vi "Main_DataSave.vi"(8 "error in":errorcluster, 11 "Queues in":T1) -> (0 "error out":errorcluster)   [LabVIEW 2019]
uses:
  Queue/TypeDef/#TypeDef_App_Queues.ctl
  User Interface/TypeDef/#TypeDef_Enum_Buttons.ctl
  User Interface/TypeDef/#TypeDef_EventStructureConstant.ctl
  User Interface/TypeDef/#TypeDef_Enum_EventStructure.ctl
  Queue/TypeDef/#TypeDef_NetworkStream.ctl
  Communication/TypeDef/#TypeDef_FromMRtoPC.ctl
  Communication/TypeDef/#TypeDef_FromPCtoMR.ctl
  Communication/TypeDef/#TypeDef_Command.ctl
  Communication/TypeDef/#TypeDef_ErrorHandler_prop.ctl
  Communication/TypeDef/#TypeDef_PropGraph.ctl
  Communication/TypeDef/#TypeDef_PropertiesToSave.ctl
  <vilib>/addons/database/Connection.llb/Conn ObjectReference.ctl
  Test/TypeDef/#TypeDef_DataToTest.ctl
  TypeDef/#TypeDef_EnumOp_DataSaving.ctl
  Communication/TypeDef/#TypeDef_SetGet.ctl
  <vilib>/event_ctls.llb/usereventprio.ctl
  <vilib>/addons/database/NI_Database_API.lvlib
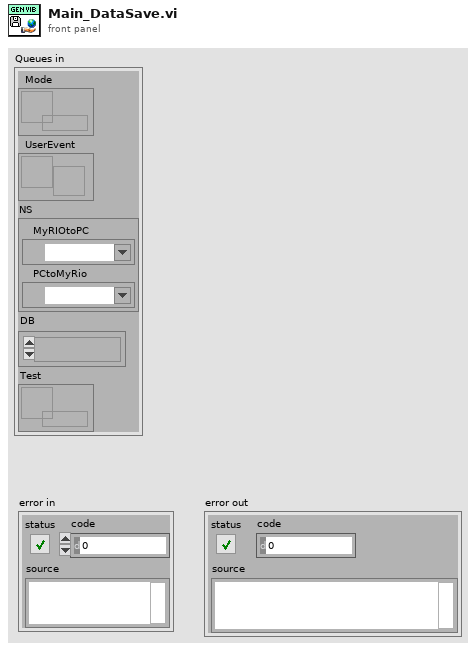
[diagram p1: front panel]
types:
  T1 = typedef "#TypeDef_App_Queues.ctl" = cluster{"Mode":refnum<queue>, "UserEvent":refnum<user-event>, "NS":T2, "DB":T3, "Test":refnum<queue>}
  T2 = typedef "#TypeDef_NetworkStream.ctl" = cluster{"MyRIOtoPC":refnum<k21>, "PCtoMyRio":refnum<k21>}
  T3 = typedef "NI_Database_API.lvlib/Conn ObjectReference.ctl" = refnum<k1>
  T4 = typedef "#TypeDef_FromMRtoPC.ctl" = cluster{"Accessibility":T5, "PropGraph":T8, "No Data?":bool, "WaveformData":waveform(dbl)[]}
  T5 = typedef "#TypeDef_FromPCtoMR.ctl" = cluster{"Command":T6, "Error?":bool, "Stop":bool, "StopPomiar":bool, "Name":string, "FilesPath":path, "ErrorHandler":T7, "Fs":dbl}
  T6 = typedef "#TypeDef_Command.ctl" = enum16{"Start", "End"}
  T7 = typedef "#TypeDef_ErrorHandler_prop.ctl" = cluster{"Threads":enum16{"Acquisistion", "Data Operation", "Save File"}, "ClearError":bool, "Error Out ":errorcluster, "Error":bool}
  T8 = typedef "#TypeDef_PropGraph.ctl" = cluster{"Raw Data":dbl[][], "Poperties":T9, "Power Spectrum / PSD":cluster{"f0":dbl, "df":dbl, "magnitude":dbl[]}[]}
  T9 = typedef "#TypeDef_PropertiesToSave.ctl" = cluster{"RMS values":dbl[], "Max":dbl[], "Min":dbl[], "A(8)":dbl[], "t":dbl, "A(8) Axis":dbl, "Aw":dbl[], "Ak 30min":dbl, "Ak_axis":i32, "Spec":cluster{"f0":dbl, "df":dbl, "magnitude":dbl[]}[]}
  T10 = typedef "#TypeDef_EnumOp_DataSaving.ctl" = enum16{"Idle", "Init", "Collecting", "Saving", "Deleting", "Error_Shutdown", "ClearError"}
  T11 = typedef "#TypeDef_SetGet.ctl" = enum16{"Set", "Get"}
  T12 = enum16{"open", "open or create", "create or replace", "create", "open (read-only)"}
  T13 = typedef "usereventprio.ctl" = enum32{"high priority", "normal priority"}
  T14 = typedef "#TypeDef_Enum_EventStructure.ctl" = enum16{"Default", "Final Items", "Moment Items", "DB"}
  T15 = typedef "#TypeDef_EventStructureConstant.ctl" = cluster{"Value":variant, "Property":T14}
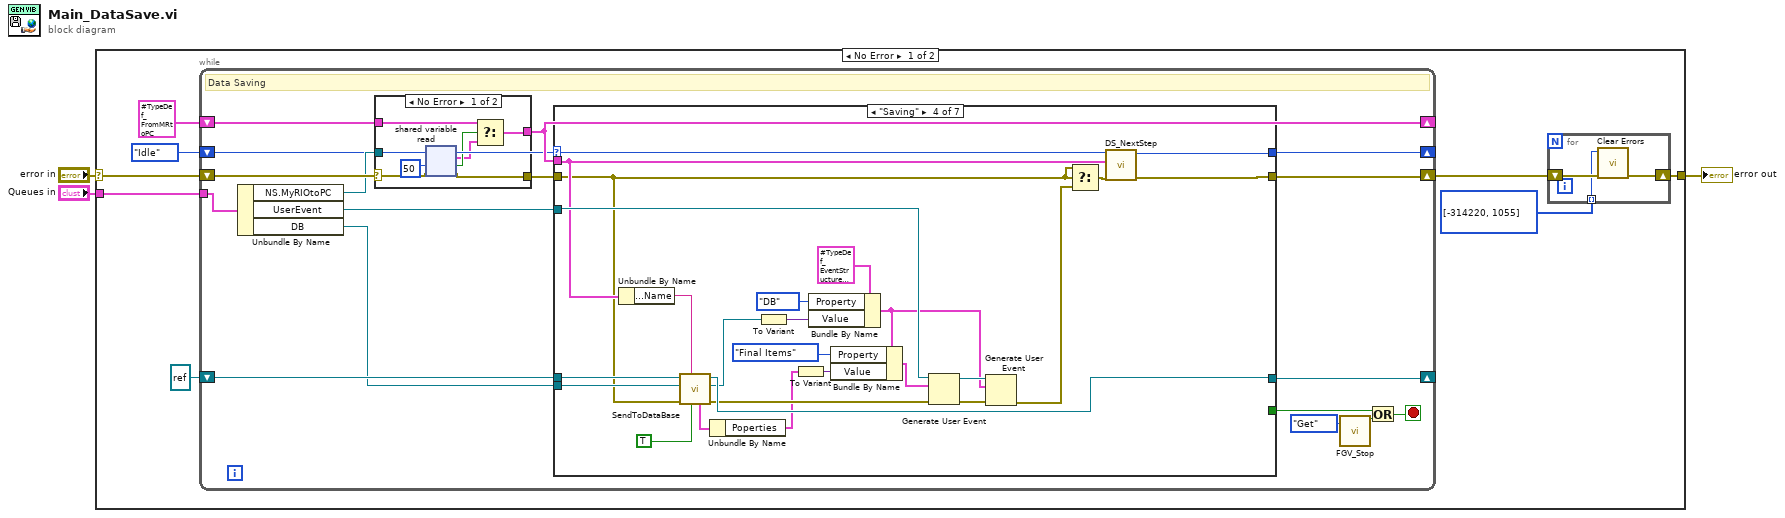
[diagram p0: block diagram]
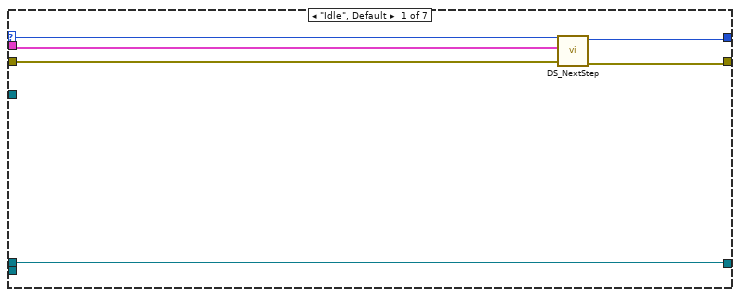
[diagram p2: hidden frame]
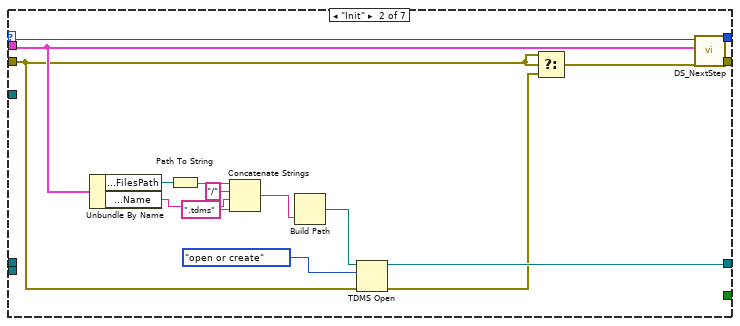
[diagram p3: hidden frame]
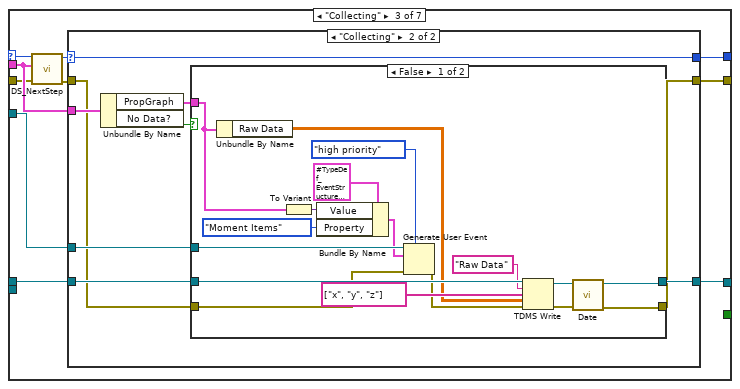
[diagram p4: hidden frame]
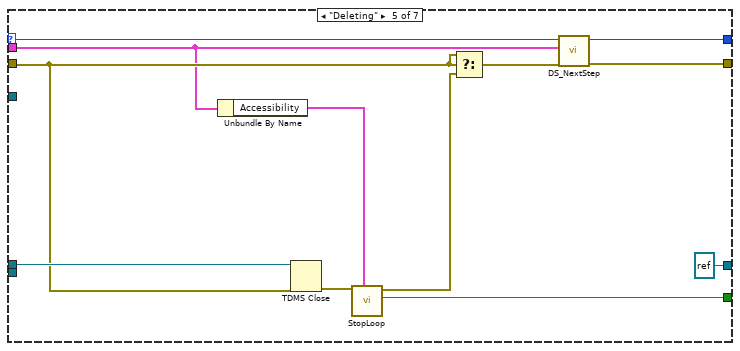
[diagram p7: hidden frame]
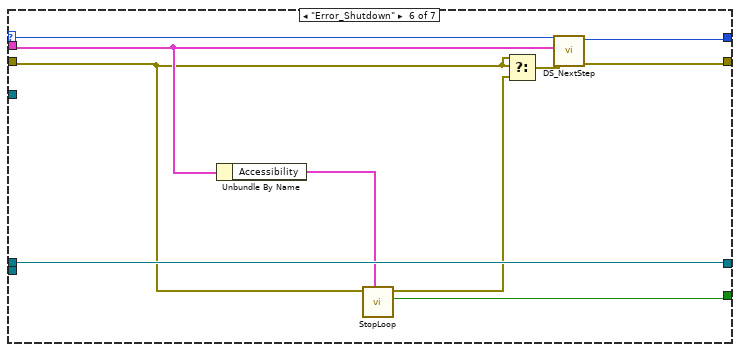
[diagram p8: hidden frame]
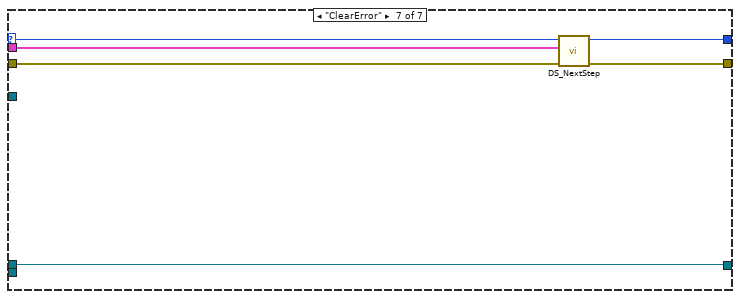
[diagram p9: hidden frame]
diagram:
  n1 = case shown="No Error" "error in" {
    selector: "error in" -> [w7 w159]
    tunnel: "Queues in" -> [w8 _]
    tunnel: [w4 w159] -> w1
    frame No Error {
      n2 = while {
        shift-right: [w26] -> w5
        shift-left: w7 -> [w31]
        shift-right: [w25] -> _
        shift-left: #TypeDef_EnumOp_DataSaving."Idle" ("EnumOp_DataAcquisition") -> [w19]
        tunnel: w8 -> [w29]
        shift-right: [w28] -> _
        shift-left: refnum<k34> refnum ("tdms file out") -> [w27]
        shift-right: [w23] -> _
        shift-left: T4 {"Accessibility"={"Command"=enum."End", "Error?"=FALSE, "Stop"=FALSE, "StopPomiar"=FALSE, "Name"="", "FilesPath"=path "", "ErrorHandler"={"Threads"=enum."Acquisistion", "ClearError"=FALSE, "Error Out "={"status"=FALSE, "code"=0, "source"=""}, "Error"=FALSE}, "Fs"=0.0}, "PropGraph"={"Raw Data"=[], "Poperties"={"RMS values"=[], "Max"=[], "Min"=[], "A(8)"=[], "t"=0.0, "A(8) Axis"=0.0, "Aw"=[], "Ak 30min"=0.0, "Ak_axis"=0, "Spec"=[]}, "Power Spectrum / PSD"=[]}, "No Data?"=FALSE, "WaveformData"=[]} ("FromMyRiOtoUI") -> [w24]
        stop <- w15 stop-if-true
        # "Data Saving"
        n3 = Unbundle By Name(w29) -> ("NS.MyRIOtoPC"=w30:refnum<k21>, "UserEvent"=w22:refnum<user-event>, "DB"=w21:T3)
        n4 = case shown="No Error" w31 {
          selector: w31 -> [w154 w158]
          tunnel: [w153 w158] -> w20
          tunnel: [w156 w157] -> w23
          tunnel: w30 -> [w150 _]
          tunnel: w24 -> [w155 w157]
          frame No Error {
            n5 = shared-variable-read(w150, w154, 50 ("timeout in ms (-1)")) -> (w153:errorcluster, w152:bool, w149:T4)  [unwired: 1 out]
            n6 = Select(t=w155, s=w152, f=w149) -> (s? t:f=w156:T4)
          }
          frame Error {
          }
        }
        n7 = case shown="\"Saving\"" w19 {
          selector: w19 -> [w35 w48 w62 w120 w127 w140 w144]
          tunnel: [w33 w53 w63 w118 refnum<k34> refnum ("tdms file out") w139 w148] -> w28
          tunnel: w27 -> [w33 _ w61 w119 w132 w139 w148]
          tunnel: [w36 w47 w56 w114 w129 w141 w146] -> w25
          tunnel: [w37 w50 w54 w98 w130 w142 w147] -> w26
          tunnel: w20 -> [w32 w44 w58 w95 w131 w134 w145]
          tunnel: w23 -> [w34 w45 w59 w115 w123 w137 w143]
          tunnel: w22 -> [_ _ w60 w117 _ _ _]
          tunnel: w21 -> [_ _ _ w116 _ _ _]
          tunnel: [_ _ _ _ w124 w138 _] -> w16
          frame "Idle", Default {
            n8 = call "DS_NextStep.vi"("error in (no error)"=w32, "FromMyRiOtoUI"=w34, "Previous step"=w35) -> ("error out"=w37:errorcluster, "Next Step"=w36:T10)  [unwired: 7 in]
          }
          frame "Init" {
            n9 = Unbundle By Name(w45) -> ("Accessibility.FilesPath"=w43:path, "Accessibility.Name"=w40:string)
            n10 = Path To String(path=w43) -> (string=w42:string)
            n11 = Concatenate Strings(w42, "/" ("string"), w40, ".tdms" ("string")) -> (w39:string)
            n12 = Build Path(name or relative path=w39) -> (appended path=w46:path)  [unwired: 1 in]
            n13 = TDMS Open(8:w44, 10:T12."open or create" ("operation (0:open)"), 11:w46) -> (0:w51:errorcluster, 3:w53:refnum<k34>)  [unwired: 4 in]
            n14 = Select(t=w44, s=w44, f=w51) -> (s? t:f=w49:errorcluster)
            n15 = call "DS_NextStep.vi"("error in (no error)"=w49, "FromMyRiOtoUI"=w45, "Previous step"=w48) -> ("error out"=w50:errorcluster, "Next Step"=w47:T10)  [unwired: 7 in]
          }
          frame "Collecting" {
            n16 = call "DS_NextStep.vi"("error in (no error)"=w58, "FromMyRiOtoUI"=w59, "Previous step"=w62) -> ("error out"=w55:errorcluster, "Next Step"=w57:T10)  [unwired: 7 in]
            n17 = case shown="\"Collecting\"" w57 {
              selector: w57 -> [w65 w70]
              tunnel: [w64 w75] -> w63
              tunnel: w61 -> [w64 w74]
              tunnel: w60 -> [_ w73]
              tunnel: w59 -> [_ w72]
              tunnel: w55 -> [w66 w71]
              tunnel: [w65 w70] -> w56
              tunnel: [w66 w69] -> w54
              frame "Saving", Default {
              }
              frame "Collecting" {
                n18 = Unbundle By Name(w72) -> ("PropGraph"=w68:T8, "No Data?"=w67:bool)
                n19 = case shown="False" w67 {
                  tunnel: [w78 w94] -> w75
                  tunnel: w74 -> [w92 w94]
                  tunnel: w73 -> [w88 _]
                  tunnel: w71 -> [w83 w93]
                  tunnel: [w76 w93] -> w69
                  tunnel: w68 -> [w81 _]
                  frame False {
                    n20 = Unbundle By Name(w81) -> ("Raw Data"=w80:dbl[][])
                    n21 = To Variant(anything=w81) -> (Variant=w84:variant)
                    n22 = Bundle By Name(cluster=T15 {"Value"=variant, "Property"=enum."Default"}, "Value"=w84, "Property"=#TypeDef_Enum_EventStructure."Moment Items") -> (w87:T15)
                    n23 = Generate User Event(priority (normal)=usereventprio."high priority", user event=w88, event data cluster=w87, error in=w83) -> (error out=w89:errorcluster)  [unwired: 1 out]
                    n24 = TDMS Write(0:w92, 5:"Raw Data" ("group name in (Untitled)"), 7:string[] ["x", "y", "z"] ("channel name(s) in (Untitled)"), 9:w80, 11:w89) -> (4:w79:refnum<k34>, 15:w77:errorcluster)  [unwired: 1 in, 2 out]
                    n25 = call "Date.vi"("error in"=w77, "Refnum in"=w79) -> ("error out"=w76:errorcluster, "Refnum out"=w78:refnum<k34>)  [unwired: 8 in]
                  }
                  frame True {
                  }
                }
              }
            }
          }
          frame "Saving" {
            n26 = Unbundle By Name(w115) -> ("Accessibility.Name"=w99:string)
            n27 = call "SendToDataBase.vi"("Put in?"=TRUE, "TableName"=w99, "error in"=w95, "Connection in"=w116, "tdms file in"=w119) -> ("error out"=w112:errorcluster, "Connection out"=w101:T3, "tdms file out"=w118:refnum<k34>, "PropGraph"=w108:T8)  [unwired: 2 in, 1 out]
            n28 = Unbundle By Name(w108) -> ("Poperties"=w107:T9)
            n29 = To Variant(anything=w101) -> (Variant=w100:variant)
            n30 = To Variant(anything=w107) -> (Variant=w111:variant)
            n31 = Bundle By Name(cluster=T15 {"Value"=variant, "Property"=enum."Default"}, "Property"=#TypeDef_Enum_EventStructure."DB", "Value"=w100) -> (w103:T15)
            n32 = Bundle By Name(cluster=w103, "Property"=#TypeDef_Enum_EventStructure."Final Items", "Value"=w111) -> (w110:T15)
            n33 = Generate User Event(user event=w117, event data cluster=w110, error in=w112) -> (user event out=w104:refnum<user-event>, error out=w106:errorcluster)  [unwired: 1 in]
            n34 = Generate User Event(user event=w104, event data cluster=w103, error in=w106) -> (error out=w97:errorcluster)  [unwired: 1 in, 1 out]
            n35 = Select(t=w95, s=w95, f=w97) -> (s? t:f=w96:errorcluster)
            n36 = call "DS_NextStep.vi"("error in (no error)"=w96, "FromMyRiOtoUI"=w115, "Previous step"=w120) -> ("error out"=w98:errorcluster, "Next Step"=w114:T10)  [unwired: 7 in]
          }
          frame "Deleting" {
            n37 = Unbundle By Name(w123) -> ("Accessibility"=w122:T5)
            n38 = TDMS Close(8:w131, 11:w132) -> (0:w126:errorcluster)  [unwired: 1 out]
            n39 = call "StopLoop.vi"("Accessibility"=w122, "error in (no error)"=w126) -> ("Stop?"=w124:bool, "error out"=w125:errorcluster)  [unwired: 8 in]
            n40 = Select(t=w131, s=w131, f=w125) -> (s? t:f=w128:errorcluster)
            n41 = call "DS_NextStep.vi"("error in (no error)"=w128, "FromMyRiOtoUI"=w123, "Previous step"=w127) -> ("error out"=w130:errorcluster, "Next Step"=w129:T10)  [unwired: 7 in]
          }
          frame "Error_Shutdown" {
            n42 = Unbundle By Name(w137) -> ("Accessibility"=w136:T5)
            n43 = call "StopLoop.vi"("Accessibility"=w136, "error in (no error)"=w134) -> ("Stop?"=w138:bool, "error out"=w135:errorcluster)  [unwired: 8 in]
            n44 = Select(t=w134, s=w134, f=w135) -> (s? t:f=w133:errorcluster)
            n45 = call "DS_NextStep.vi"("error in (no error)"=w133, "FromMyRiOtoUI"=w137, "Previous step"=w140) -> ("error out"=w142:errorcluster, "Next Step"=w141:T10)  [unwired: 7 in]
          }
          frame "ClearError" {
            n46 = call "DS_NextStep.vi"("error in (no error)"=w145, "FromMyRiOtoUI"=w143, "Previous step"=w144) -> ("error out"=w147:errorcluster, "Next Step"=w146:T10)  [unwired: 7 in]
          }
        }
        n47 = call "FGV_Stop.vi"("Get/Set"=#TypeDef_SetGet."Get") -> ("STOP out"=w18:bool)  [unwired: 10 in]
        n48 = Or(x=w16, y=w18) -> (x .or. y?=w15:bool)
      }
      n49 = for {
        shift-right: [w13] -> w4
        shift-left: w5 -> [w14]
        tunnel: i32[] [-314220, 1055] -> [w12] mode=indexing
        n50 = call <vilib>:"Clear Errors.vi"("error in (no error)"=w14, "specific error code to clear (0: all)"=w12) -> ("error out"=w13:errorcluster)  [unwired: 4 in, 1 out]
      }
    }
    frame Error {
    }
  }
  "error out" <- w1
